vi "Cleanup.vi"(8 "error in (no error)":errorcluster) -> (0 "error out":errorcluster)   [LabVIEW 2017, in "Front Panel Publisher.lvlib" / "Websocket.lvclass"]
uses:
  Websocket.lvclass
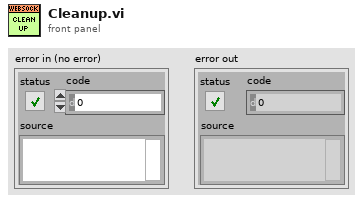
[diagram p1: front panel]
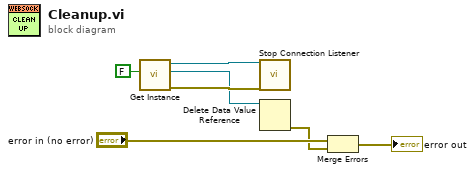
[diagram p0: block diagram]
diagram:
  n1 = call "Get Instance.vi"("Create If Not Exist (T)"=FALSE) -> ("error out"=w4:errorcluster, "DVRRefOut"=w2:refnum<data-value>, "WebSocket Out"=w3:refnum<class "Websocket.lvclass">)  [unwired: 6 in, 2 out]
  n2 = call "Stop Connection Listener.vi"("Websocket In"=w3, "error in (no error)"=w4) -> ()  [unwired: 16 in, 2 out]
  n3 = Delete Data Value Reference(data value reference=w2) -> (error out=w5:errorcluster)  [unwired: 1 in, 1 out]
  n4 = Merge Errors("error in (no error)", w5) -> (→"error out":errorcluster)
